vi "PowerIn MSMT Get Measure Step from DB.vi"(8 "error in (no error)":errorcluster, 10 "Standard":string, 11 "Servo MSMT in":refnum<class "Input Power Measurement.lvclass">) -> (0 "error out":errorcluster, 2 "Step Out":refnum<k7>, 3 "Servo MSMT out":refnum<class "Input Power Measurement.lvclass">)   [LabVIEW 2014, in "Input Power Measurement.lvclass"]
uses:
  Input Power Measurement.lvclass
  QPA Measurement/QPA Measurement.lvlibp/Sequence Automation/Classes/QPA Measurement/Protected Methods/Read Measurement Name.vi
  QPA Measurement/QPA Measurement.lvlibp/Sequence Automation/Classes/QPA Measurement/QPA Measurement.lvclass
  TestStand API Tools/Step Actions/TSAT Step Actions.lvlib
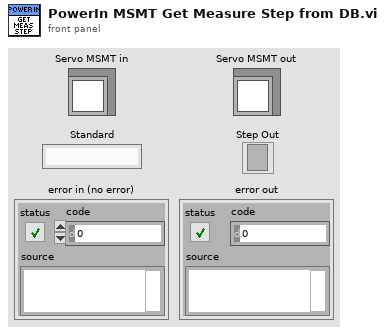
[diagram p1: front panel]
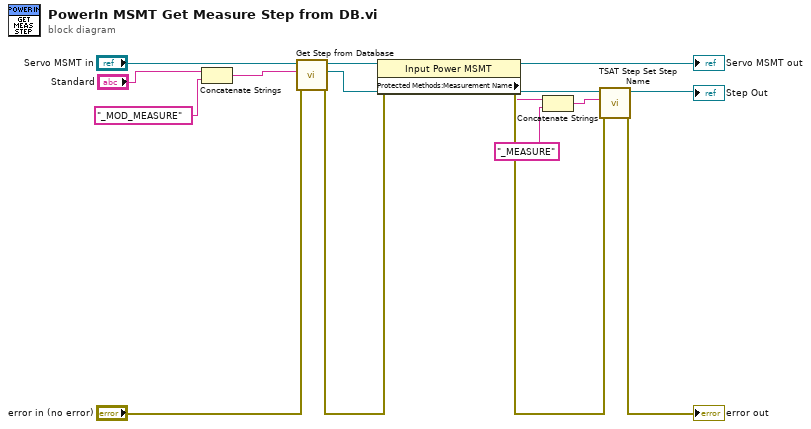
[diagram p0: block diagram]
diagram:
  n1 = Concatenate Strings("Standard", "_MOD_MEASURE" ("string")) -> (w2:string)
  n2 = call "Get Step from Database.vi"("error in (no error)"="error in (no error)", "Default Step"=w2, "QPA Measurement in"="Servo MSMT in") -> ("error out"=w10:errorcluster, "Step Out"=w13:refnum<k7>, "QPA Measurement out"=w7:refnum<class "Input Power Measurement.lvclass">)  [unwired: 6 in]
  n3 = property class="Input Power MSMT"(reference=w7, error in=w10) -> (reference out=→"Servo MSMT out":refnum<class "Input Power Measurement.lvclass">, error out=w8:errorcluster, "Protected Methods:Measurement Name"=w5:string)
  n4 = Concatenate Strings(w5, "_MEASURE" ("string")) -> (w4:string)
  n5 = call "TSAT Step Set Step Name.vi"("Error In"=w8, "Name"=w4, "Step In"=w13) -> ("Error Out"=→"error out":errorcluster, "Step Out"=→"Step Out":refnum<k7>)  [unwired: 7 in]
